vi "禹山电导率_获取温度和测量值.vi"(8 "error in (no error)":errorcluster caption="错误输入（无错误）", 11 "MB session in":refnum<class "MB_Master.lvclass">) -> (0 "error out":errorcluster caption="错误输出", 2 "输出值":cluster{"温度测量值":sgl, "电导率":sgl, "错误标志":u16} {"错误标志" items=["NO Error"=0, "量程切换错误标识"=255]}, 3 "MB session out":refnum<class "MB_Master.lvclass">)   [LabVIEW 2016, in "斯坦道多参数.lvlib"]
uses:
  <vilib>/Plasmionique/MB Master/MB_Master/MB_Master.lvclass
  <vilib>/Plasmionique/MB Master/MB Master.lvlib
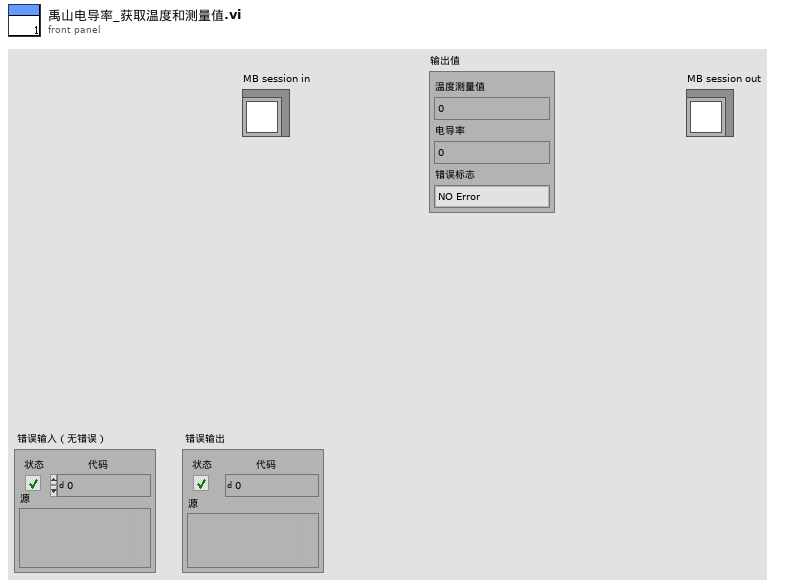
[diagram p1: front panel]
types:
  T1 = cluster{"pH":u32, "DO":u32, "Cond":u32, "Turb":u32, "叶绿素a":u32, "藻密度":u32, "ORP":u32}
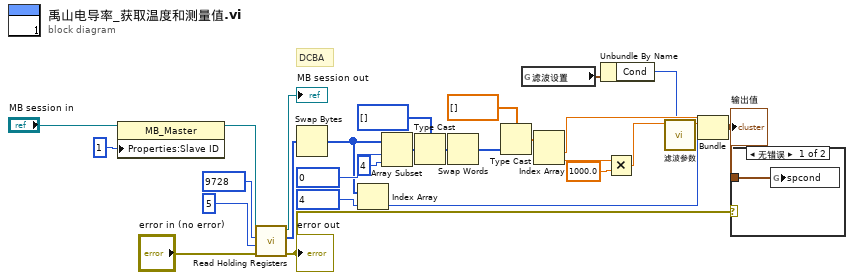
[diagram p0: block diagram]
diagram:
  # "DCBA"
  n1 = property class="MB_Master"(reference="MB session in", "Properties:Slave ID"=u16 1 ("y")) -> (reference out=w20:refnum<class "MB_Master.lvclass">)  [unwired: 1 in, 1 out]
  n2 = call <vilib>:"Read Holding Registers.vi"("error in (no error)"="error in (no error)", "quantity"=u16 5, "starting address"=u16 9728, "MB session in"=w20) -> ("error out"=w14:errorcluster, "Registers"=w18:u16[], "MB session out"=→"MB session out":refnum<class "MB_Master.lvclass">)  [unwired: 5 in]
  "error out" <- w14
  n3 = Swap Bytes(anything=w18) -> (byte swapped=w8:u16[])
  n4 = Index Array(array=w8, index=u16 4 ("starting address")) -> (element=w7:u16)
  n5 = Array Subset(array=w8, index=u16 0 ("starting address"), length=4 ("长度")) -> (w12:u16[])
  n6 = Type Cast(type=u32[] [] ("数组 2"), x=w12) -> (*(type *) &x=w24:u32[])
  n7 = Swap Words(1:w24) -> (0:w26:u32[])
  n8 = Type Cast(type=sgl[] [] ("数组 2"), x=w26) -> (*(type *) &x=w22:sgl[])
  n9 = global read "断电保存变量.vi" "滤波设置"() -> (w2:T1)
  n10 = Index Array(array=w22) -> (element #1=w17:sgl, element #2=w16:sgl)  [unwired: 2 in]
  n11 = Unbundle By Name(w2) -> ("Cond"=w1:u32)
  n12 = Multiply(x=w16, y=sgl 1000.0) -> (x*y=w4:sgl)
  n13 = call "滤波参数.vi"("滤波次数"=w1, "x"=w4) -> ("mode"=w3:dbl)  [unwired: 9 in]
  n14 = Bundle("数值"=w17, "mode"=w3, w7) -> (w13:cluster{"数值":sgl, "mode":dbl, u16})  [unwired: 1 in]
  "输出值" <- w13
  n15 = case shown="无错误" w14 {
    tunnel: w13 -> [w29 _]
    frame No Error {
      n16 = global write "禹山过程全局变量.vi" "spcond"(w29) -> ()
    }
    frame Error {
    }
  }
